vi "Create Object Dependency.vi"(10 "Error In":errorcluster, 11 "Dependency Properties":T1) -> (2 "Error Out":errorcluster, 3 "Dependency .NET Ref Out":refnum<k24>)   [LabVIEW 2015, in "VeriStand Custom Device XML Parser.lvlib"]
doc: "Creates a dependency object based on the provided properties"
uses:
  VeriStand Custom Device XML Parser.lvlib
  NationalInstruments.VeriStand.XMLReader
  XML Controls/Dependency Properties.ctl
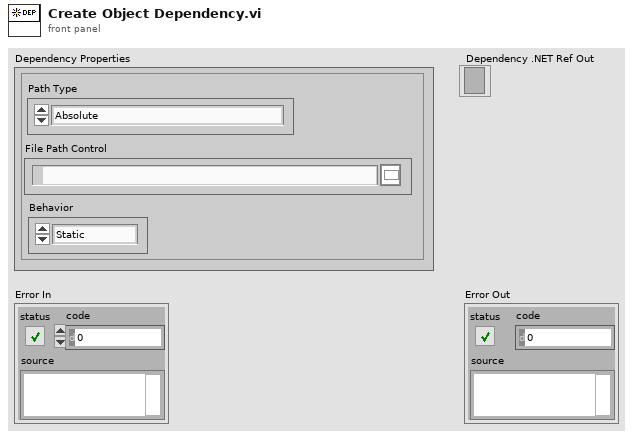
[diagram p1: front panel]
types:
  T1 = typedef "VeriStand Custom Device XML Parser.lvlib/Dependency Properties.ctl" = cluster{"File Path Control":path, "Path Type":enum16{"Absolute", "To Base", "To Common Doc Dir", "To Application Data Dir"}, "Behavior":enum16{"Static", "Dynamic"}}
  T2 = enum16{"Absolute", "To Base", "To Common Doc Dir", "To Application Data Dir"}
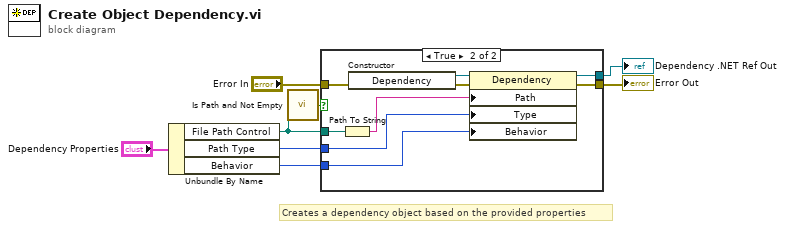
[diagram p0: block diagram]
diagram:
  # "Creates a dependency object based on the provided properties"
  n1 = Unbundle By Name("Dependency Properties") -> ("File Path Control"=w4:path, "Path Type"=w5:T2, "Behavior"=w6:enum16{"Static", "Dynamic"})
  n2 = call <vilib>:"Is Path and Not Empty.vi"("path"=w4) -> ("Is Path and Not Empty?"=w2:bool)  [unwired: 4 in]
  n3 = case shown="True" w2 {
    tunnel: "Error In" -> [w9 w18]
    tunnel: w4 -> [_ w15]
    tunnel: w5 -> [_ w13]
    tunnel: w6 -> [_ w12]
    tunnel: [_ w11] -> w8
    tunnel: [w9 w10] -> w7
    frame False {
    }
    frame True {
      n4 = Path To String(path=w15) -> (string=w14:string)
      n5 = constructor class="Dependency"(error in=w18) -> (reference out=w16:refnum<k24>, error out=w17:errorcluster)  [unwired: 2 in, 1 out]
      n6 = property class="Dependency"(reference=w16, error in=w17, "Path"=w14, "Type"=w13, "Behavior"=w12) -> (reference out=w11:refnum<k24>, error out=w10:errorcluster)
    }
  }
  "Dependency .NET Ref Out" <- w8
  "Error Out" <- w7
